vi "Enum Value.vi"(10 "Enumeration":T1) -> (2 "Value":i32)   [LabVIEW 2020, in "Enum Template.lvlib"]
uses:
  Enumeration.ctl
  Enum Template.lvlib
  proto/hello/lv/TestEnum/TestEnum.lvlib
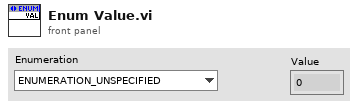
[diagram p1: front panel]
types:
  T1 = typedef "TestEnum.lvlib/Enumeration.ctl" = enum16{"ENUMERATION_UNSPECIFIED"}
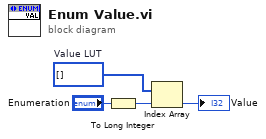
[diagram p0: block diagram]
diagram:
  w4 = i32[] []  # Value LUT
  n1 = To Long Integer(number="Enumeration") -> (32bit integer=w1:i32)
  n2 = Index Array(array=w4, index=w1) -> (element=→"Value":i32)
